vi "Set Format.vi"(8 "error in (no error)":errorcluster, 9 "format (0 : log mag)":u16(ring) items=["log magnitude", "phase", "delay", "Smith chart", "polar", "linear magnitude", "standing wave ratio", "real", "imaginary"], 11 "VISA resource name":refnum<visa-resource-name>) -> (0 "error out":errorcluster, 3 "VISA resource name out":refnum<visa-resource-name>)   [LabVIEW 2018, in "Agilent 87XX Series.lvlib"]
doc: "This VI for the HP8753B is used to set the meausurement format."
uses:
  Agilent 87XX Series.lvlib
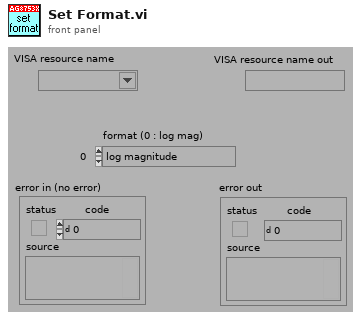
[diagram p1: front panel]
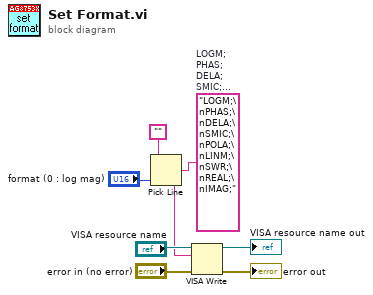
[diagram p0: block diagram]
diagram:
  w5 = "LOGM;\nPHAS;\nDELA;\nSMIC;\nPOLA;\nLINM;\nSWR;\nREAL;\nIMAG;"  # LOGM; PHAS; DELA; SMIC; POLA; LINM; SWR; REAL; IMAG;
  n1 = Pick Line(string ("")="", multi-line string=w5, line index="format (0 : log mag)") -> (output string=w1:string)
  n2 = VISA Write(VISA resource name="VISA resource name", write buffer=w1, error in (no error)="error in (no error)") -> (VISA resource name out=→"VISA resource name out":refnum<visa-resource-name>, error out=→"error out":errorcluster)  [unwired: 1 out]
